vi "QD_Washing_Machine.vi"(0 "Data_In":T1, 1 "Max_Queue_Size_In":i32=-1, 2 "Queue_Name_In":string, 5 "Data_In":T1[](array[typedef]), 7 "Time_Out_In_ms (-1)":i32, 11 "Error_In":errorcluster, 13 "Queue_Operation_Select":T2=enum."Enqueue") -> (4 "Data_Out":T1, 6 "Total_Data":T1[](array[typedef]), 15 "Error_Out":errorcluster)   [LabVIEW 2023]
doc: "Used to send the state and event data from one state to another"
uses:
  Controls/Queue_Operation_Select.ctl
  Controls/State_and_Data.ctl
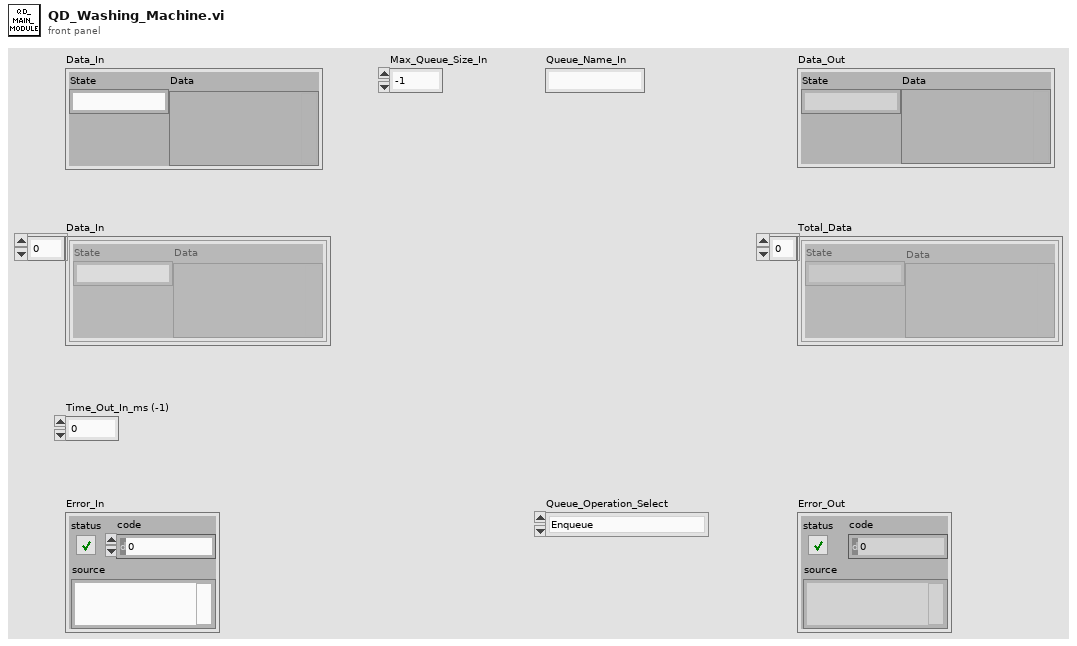
[diagram p1: front panel]
types:
  T1 = typedef "State_and_Data.ctl" = cluster{"State":string, "Data":variant}
  T2 = typedef "Queue_Operation_Select.ctl" = enum16{"Obtain_Queue", "Enqueue", "Enqueue_First", "Enqueue_N", "Lossy_Enqueue", "Preview", "Queue_Status", "Dequeue", "Flush", "Release_Queue"}
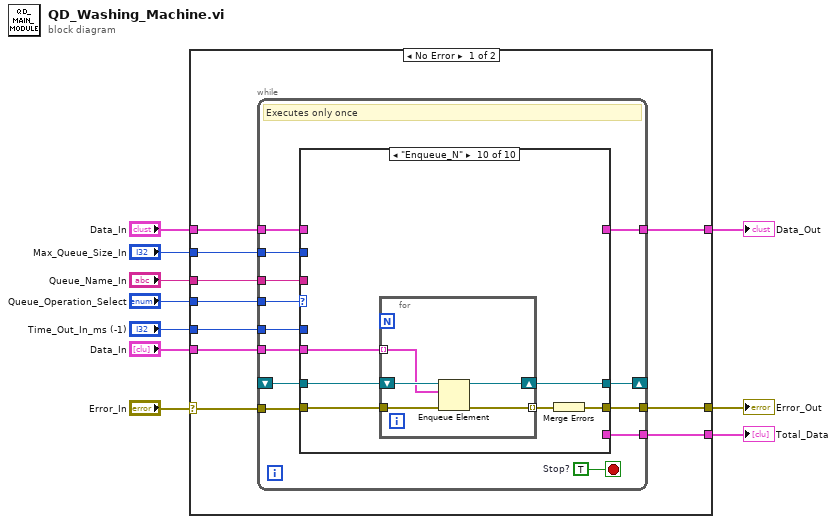
[diagram p0: block diagram]
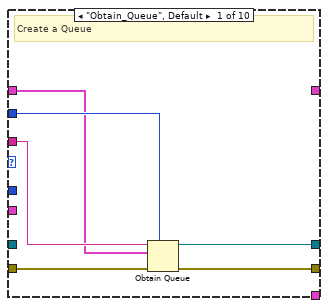
[diagram p2: hidden frame]
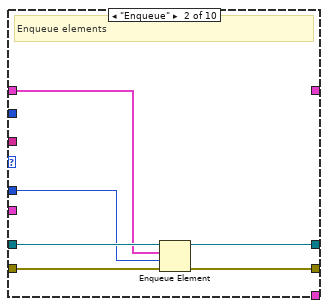
[diagram p3: hidden frame]
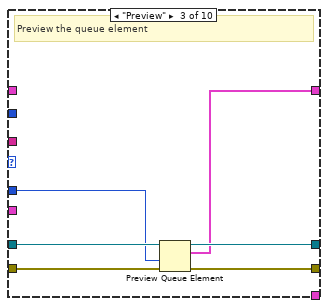
[diagram p4: hidden frame]
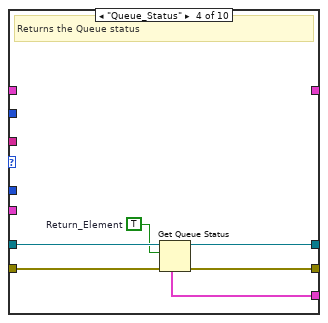
[diagram p5: hidden frame]
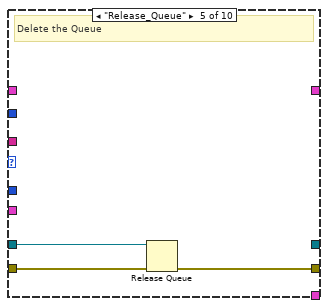
[diagram p6: hidden frame]
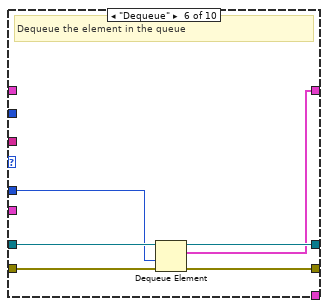
[diagram p7: hidden frame]
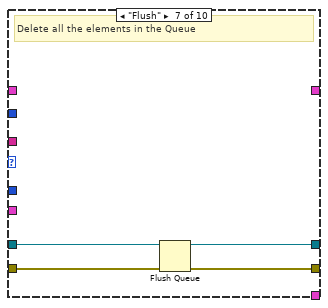
[diagram p8: hidden frame]
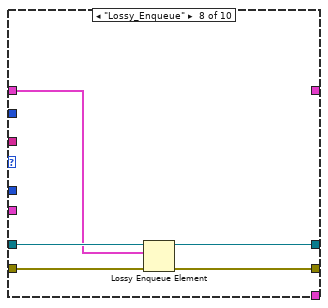
[diagram p9: hidden frame]
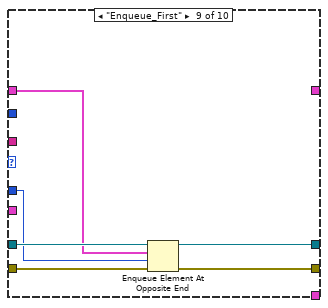
[diagram p10: hidden frame]
diagram:
  n1 = case shown="No Error" "Error_In" {
    selector: "Error_In" -> [w12 w93]
    tunnel: "Max_Queue_Size_In" -> [w20 _]
    tunnel: [w19 w93] -> w9
    tunnel: "Data_In" -> [w18 _]
    tunnel: "Time_Out_In_ms (-1)" -> [w17 _]
    tunnel: [w16 _] -> w6
    tunnel: "Queue_Operation_Select" -> [w15 _]
    tunnel: "Queue_Name_In" -> [w14 _]
    tunnel: [w13 _] -> w3
    tunnel: "Data_In" -> [w11 _]
    frame No Error {
      n2 = while {
        tunnel: w20 -> [w33]
        tunnel: w17 -> [w30]
        tunnel: w15 -> [w27]
        tunnel: [w25] -> w13
        shift-right: [w28] -> _
        shift-left: _ -> [w23]
        tunnel: w12 -> [w24]
        tunnel: [w32] -> w19
        tunnel: w18 -> [w31]
        tunnel: [w29] -> w16
        tunnel: w14 -> [w26]
        tunnel: w11 -> [w21]
        stop <- w22 stop-if-true
        w22 = TRUE  # Stop?
        # "Executes only once"
        n3 = case shown="\"Enqueue_N\"" w27 {
          tunnel: w24 -> [w39 w45 w50 w56 w59 w65 w69 w74 w81 w87]
          tunnel: w26 -> [w37 _ _ _ _ _ _ _ _ _]
          tunnel: w33 -> [w36 _ _ _ _ _ _ _ _ _]
          tunnel: [w34 w41 w49 w55 _ w64 w68 w73 w78 w83] -> w28
          tunnel: [w38 w44 w48 w54 w58 w62 w67 w72 w80 w85] -> w32
          tunnel: w23 -> [_ w43 w51 w57 w60 w66 w70 w75 w79 w84]
          tunnel: w31 -> [w35 w42 _ _ _ _ _ w71 w77 _]
          tunnel: w30 -> [_ w40 w47 _ _ w61 _ _ w76 _]
          tunnel: [_ _ w46 _ _ w63 _ _ _ _] -> w29
          tunnel: [_ _ _ w53 _ _ _ _ _ _] -> w25
          tunnel: w21 -> [_ _ _ _ _ _ _ _ _ w82]
          frame "Obtain_Queue", Default {
            # "Create a Queue"
            n4 = Obtain Queue(max queue size (-1, unlimited)=w36, name (unnamed)=w37, element data type=w35, error in (no error)=w39) -> (queue out=w34:refnum<queue>, error out=w38:errorcluster)  [unwired: 1 in, 1 out]
          }
          frame "Enqueue" {
            # "Enqueue elements"
            n5 = Enqueue Element(queue=w43, element=w42, timeout in ms (-1)=w40, error in (no error)=w45) -> (queue out=w41:refnum<queue>, error out=w44:errorcluster)  [unwired: 1 out]
          }
          frame "Preview" {
            # "Preview the queue element"
            n6 = Preview Queue Element(queue=w51, timeout in ms (-1)=w47, error in (no error)=w50) -> (queue out=w49:refnum<queue>, element=w46:T1, error out=w48:errorcluster)  [unwired: 1 out]
          }
          frame "Queue_Status" {
            w52 = TRUE  # Return_Element
            # "Returns the Queue status"
            n7 = Get Queue Status(queue=w57, return elements? (F)=w52, error in (no error)=w56) -> (queue out=w55:refnum<queue>, error out=w54:errorcluster, elements=w53:T1[])  [unwired: 5 out]
          }
          frame "Release_Queue" {
            # "Delete the Queue"
            n8 = Release Queue(queue=w60, error in (no error)=w59) -> (error out=w58:errorcluster)  [unwired: 1 in, 2 out]
          }
          frame "Dequeue" {
            # "Dequeue the element in the queue"
            n9 = Dequeue Element(queue=w66, timeout in ms (-1)=w61, error in (no error)=w65) -> (queue out=w64:refnum<queue>, element=w63:T1, error out=w62:errorcluster)  [unwired: 1 out]
          }
          frame "Flush" {
            # "Delete all the elements in the Queue"
            n10 = Flush Queue(queue=w70, error in (no error)=w69) -> (queue out=w68:refnum<queue>, error out=w67:errorcluster)  [unwired: 1 out]
          }
          frame "Lossy_Enqueue" {
            n11 = Lossy Enqueue Element(queue=w75, element=w71, error in (no error)=w74) -> (queue out=w73:refnum<queue>, error out=w72:errorcluster)  [unwired: 2 out]
          }
          frame "Enqueue_First" {
            n12 = Enqueue Element At Opposite End(queue=w79, element=w77, timeout in ms (-1)=w76, error in (no error)=w81) -> (queue out=w78:refnum<queue>, error out=w80:errorcluster)  [unwired: 1 out]
          }
          frame "Enqueue_N" {
            n13 = for {
              tunnel: w87 -> [w92]
              tunnel: [w91] -> w86 mode=indexing
              shift-right: [w89] -> w83
              shift-left: w84 -> [w90]
              tunnel: w82 -> [w88] mode=indexing
              n14 = Enqueue Element(queue=w90, element=w88, error in (no error)=w92) -> (queue out=w89:refnum<queue>, error out=w91:errorcluster)  [unwired: 1 in, 1 out]
            }
            n15 = Merge Errors(w86) -> (w85:errorcluster)
          }
        }
      }
    }
    frame Error {
    }
  }
  "Error_Out" <- w9
  "Data_Out" <- w6
  "Total_Data" <- w3
